vi "Look down.vi"(8 "column":i32, 9 "row":i32, 10 "Tree":T1, 11 "Array":T1[][](array[typedef])) -> (2 "output cluster":T1)   [LabVIEW 2020]
uses:
  tree--cluster.ctl
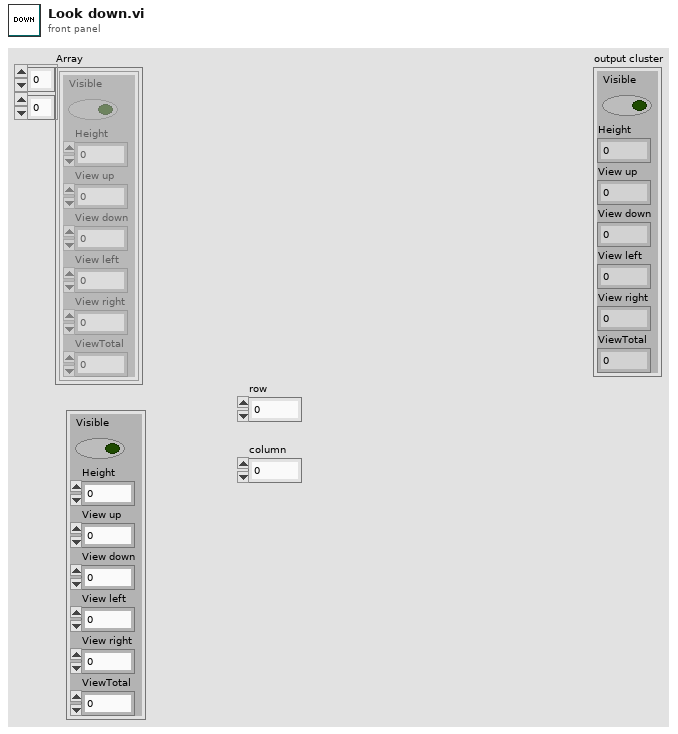
[diagram p1: front panel]
types:
  T1 = typedef "tree--cluster.ctl" = cluster{"Visible":bool, "Height":i32, "View up":i32, "View down":i32, "View left":i32, "View right":i32, "ViewTotal":i32}
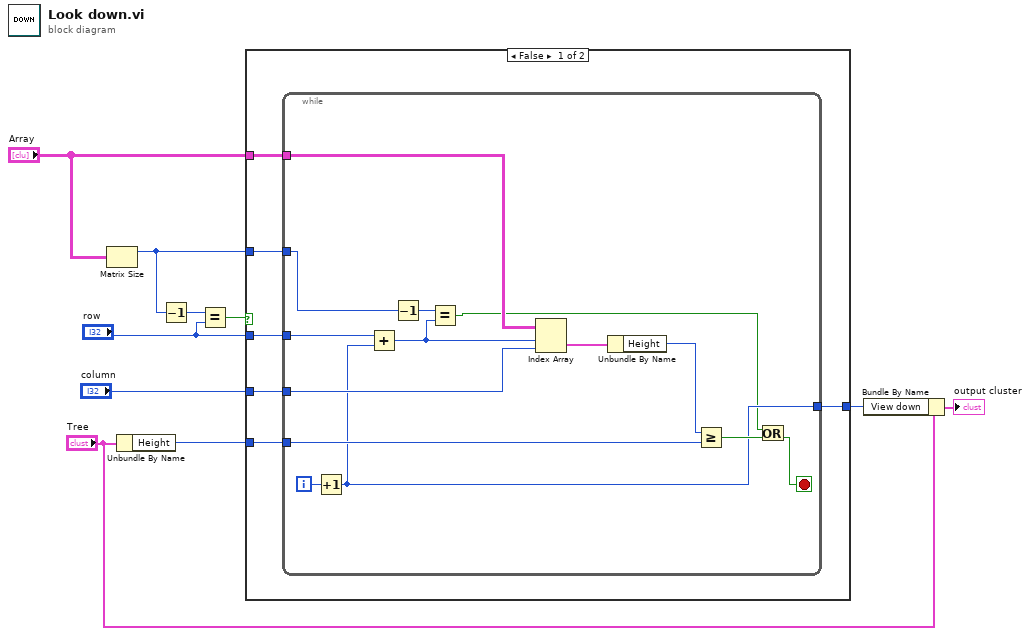
[diagram p0: block diagram]
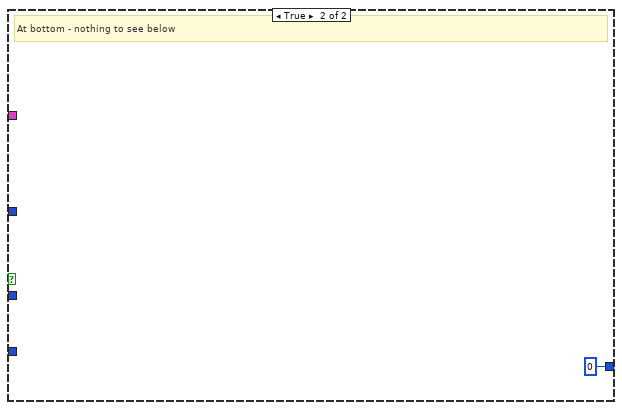
[diagram p2: hidden frame]
diagram:
  n1 = Matrix Size(0:"Array") -> (1:w3:i32)  [unwired: 1 out]
  n2 = Unbundle By Name("Tree") -> ("Height"=w10:i32)
  n3 = Decrement(x=w3) -> (x-1=w4:i32)
  n4 = Equal?(x=w4, y="row") -> (x = y?=w2:bool)
  n5 = case shown="False" w2 {
    tunnel: w10 -> [w16 _]
    tunnel: "column" -> [w15 _]
    tunnel: "row" -> [w14 _]
    tunnel: [w13 0] -> w7
    tunnel: "Array" -> [w12 _]
    tunnel: w3 -> [w11 _]
    frame False {
      n6 = while {
        tunnel: w16 -> [w24]
        tunnel: w12 -> [w30]
        tunnel: w15 -> [w29]
        tunnel: w14 -> [w28]
        tunnel: [w22] -> w13
        tunnel: w11 -> [w19]
        i -> [w27]
        stop <- w18 stop-if-true
        n7 = Increment(x=w27) -> (x+1=w22:i32)
        n8 = Add(x=w28, y=w22) -> (x+y=w21:i32)
        n9 = Decrement(x=w19) -> (x-1=w20:i32)
        n10 = Equal?(x=w20, y=w21) -> (x = y?=w17:bool)
        n11 = Index Array(array=w30, index (row)=w21, index (col)=w29) -> (element=w26:T1)
        n12 = Unbundle By Name(w26) -> ("Height"=w25:i32)
        n13 = Greater Or Equal?(x=w25, y=w24) -> (x >= y?=w23:bool)
        n14 = Or(x=w17, y=w23) -> (x .or. y?=w18:bool)
      }
    }
    frame True {
      # "At bottom - nothing to see below"
    }
  }
  n15 = Bundle By Name(cluster="Tree", "View down"=w7) -> (→"output cluster":T1)
